vi "testAppendErrorInformation_Warning_withoutState.vi"(8 "error in (no error)":errorcluster, 11 "testStateMachineUtilities in":refnum<class "testStateMachineUtilities.lvclass">) -> (0 "error out":errorcluster, 3 "testStateMachineUtilities out":refnum<class "testStateMachineUtilities.lvclass">)   [LabVIEW 2013, in "testStateMachineUtilities.lvclass"]
uses:
  testStateMachineUtilities.lvclass
  source/State Machine Support API/Parse State Queue_2024.vi
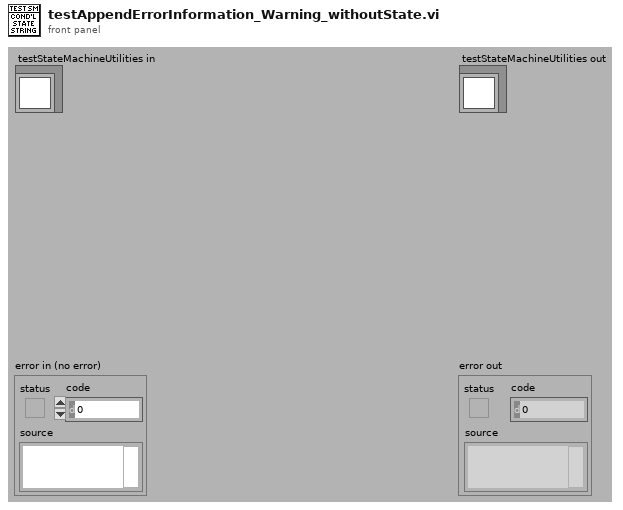
[diagram p1: front panel]
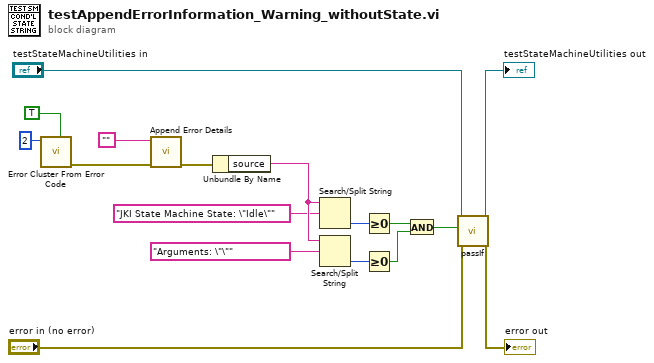
[diagram p0: block diagram]
diagram:
  n1 = call <vilib>:"Error Cluster From Error Code.vi"("is warning? (False)"=TRUE, "error code (0)"=2) -> ("error out"=w8:errorcluster)  [unwired: 7 in]
  n2 = call "Append Error Details.vi"("error in (no error)"=w8, "Previous State and Argument(s)"="") -> ("error out"=w7:errorcluster)  [unwired: 9 in]
  n3 = Unbundle By Name(w7) -> ("source"=w6:string)
  n4 = Search/Split String(string=w6, search string/char (-)="JKI State Machine State: \"Idle\"") -> (offset of match=w13:i32)  [unwired: 1 in, 2 out]
  n5 = Search/Split String(string=w6, search string/char (-)="Arguments: \"\"") -> (offset of match=w12:i32)  [unwired: 1 in, 2 out]
  n6 = Greater Or Equal To 0?(x=w13) -> (x >= 0?=w11:bool)
  n7 = Greater Or Equal To 0?(x=w12) -> (x >= 0?=w10:bool)
  n8 = And(x=w11, y=w10) -> (x .and. y?=w5:bool)
  n9 = call-dynamic "passIf.vi"("error in (no error)"="error in (no error)", "pass"=w5, "TestCase in"="testStateMachineUtilities in") -> ("error out"=→"error out":errorcluster, "TestCase out"=→"testStateMachineUtilities out":refnum<class "testStateMachineUtilities.lvclass">)  [unwired: 7 in]
